vi "WriteOutbitsGlobalVars.vi"(0 "writeState":bool, 1 "OutBitsState":T1, 2 "write_OutBitStopListening":bool, 3 "OutBitStopListening":bool, 10 "nOfCmdsOutbit0":u32, 12 "nOfCmdsOutbit1":u32, 14 "nOfCmdsOutbit2":u32, 16 "write_nOfCmdsOutbitsAll":bool) -> ()   [LabVIEW 2014]
uses:
  OutbitsStateControl.ctl
  <vilib>/rvi/Emulation/niFpgaSctlEmulationGetInTimedLoop.vi
  OutbitsGlobalVars.vi
  <vilib>/rvi/Emulation/niFpgaProcessEmulError.vi
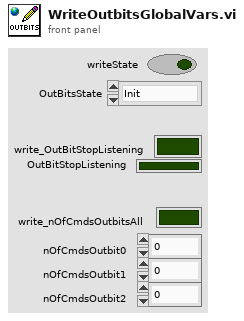
[diagram p1: front panel]
types:
  T1 = typedef "OutbitsStateControl.ctl" = enum16{"Init", "Idle", "loading", "listening", "clearing", "error"}
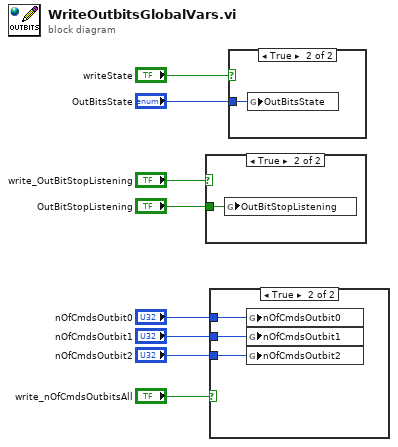
[diagram p0: block diagram]
diagram:
  n1 = case shown="True" "write_OutBitStopListening" {
    tunnel: "OutBitStopListening" -> [_ w9]
    frame False {
    }
    frame True {
      n2 = global write "OutbitsGlobalVars.vi" "OutBitStopListening"(w9) -> ()
    }
  }
  n3 = case shown="True" "write_nOfCmdsOutbitsAll" {
    tunnel: "nOfCmdsOutbit0" -> [_ w12]
    tunnel: "nOfCmdsOutbit1" -> [_ w11]
    tunnel: "nOfCmdsOutbit2" -> [_ w10]
    frame False {
    }
    frame True {
      n4 = global write "OutbitsGlobalVars.vi" "nOfCmdsOutbit0"(w12) -> ()
      n5 = global write "OutbitsGlobalVars.vi" "nOfCmdsOutbit1"(w11) -> ()
      n6 = global write "OutbitsGlobalVars.vi" "nOfCmdsOutbit2"(w10) -> ()
    }
  }
  n7 = case shown="True" "writeState" {
    tunnel: "OutBitsState" -> [_ w13]
    frame False {
    }
    frame True {
      n8 = global write "OutbitsGlobalVars.vi" "OutBitsState"(w13) -> ()
    }
  }
